vi "licdf get serial.vi"(8 "error in (no error)":errorcluster, 9 "out_size":i32, 10 "out":string, 11 "handle":i32) -> (0 "error out":errorcluster, 2 "out out":string, 3 "function return":i32)   [LabVIEW 2026, in "keynub_licdongle.lvlib"]
doc: "int32_t licdf_get_serial(int32_t handle, char *out, int32_t out_size);"
uses:
  keynub_licdongle.lvlib
  natives/win-x64/keynub_licdongle_flat.dll
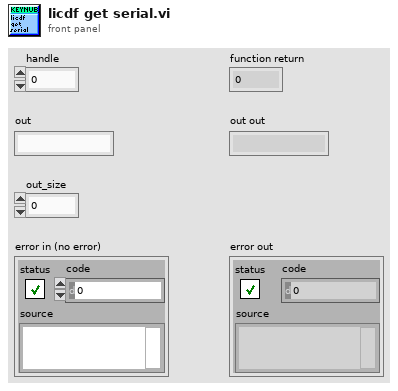
[diagram p1: front panel]
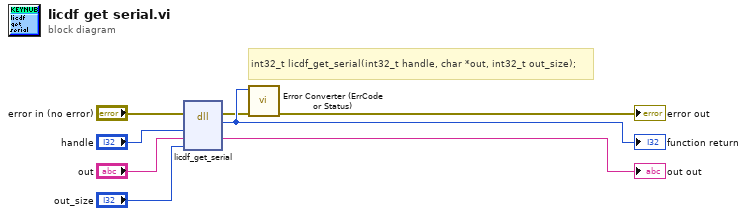
[diagram p0: block diagram]
diagram:
  # "int32_t licdf_get_serial(int32_t handle, char *out, int32_t out_size);"
  n1 = dll-call lib="C:/Austausch/KeyNub/LicenseDongle-PublicSDK/natives/win-x64/keynub_licdongle_flat.*" fn="licdf_get_serial"(error in="error in (no error)", "handle"="handle", "out"="out", "out_size"="out_size") -> (error out=w2:errorcluster, w8:i32, "out"=→"out out":string)  [unwired: 4 in, 1 out]
  "function return" <- w8
  n2 = call "Error Converter (ErrCode or Status).vi"("error in (no error)"=w2, "error code"=w8) -> ("error out"=→"error out":errorcluster)  [unwired: 9 in]
